vi "Named Controls Test.vi"() -> ()   [LabVIEW 2013]
uses:
  Dashboard Code/Preferences/Named Control.ctl
  Common Code/Dashboard UDP Packet.ctl
  Common Code/Dashboard UDP/Camera Controls.ctl
  Common Code/Dashboard UDP/Gyro Controls.ctl
  Common Code/Dashboard UDP/PID Params.ctl
  Common Code/Dashboard UDP/Encoder Controls.ctl
  Common Code/Dashboard UDP/Auto Shift Controls.ctl
  Common Code/Dashboard UDP/Auton Controls.ctl
  Common Code/Dashboard UDP/Shooter Controls.ctl
  Common Code/Dashboard UDP/Roller Controls.ctl
panel:
  out "Count":i32
  out "Names List":string[](array[string])
  in  "Page Index (-1 = All)":i32=-1
  out "Warnings List":string
  out "Named Controls":T1
  in  "Tab Control":enum32{"Page 0", "Page 1", "Page 2"}(tab)
  in  "Color Components":T2={"Hue"={110.0, 142.0}, "Sat"={138.0, 255.0}, "Val"={139.0, 198.0}} {"Val" scale=0.0..255.0; "Sat" scale=0.0..255.0; "Hue" scale=0.0..255.0 scale format="%#_3g"}
  in  "UDP Packet":T3={"Camera"={"Camera/View Angle X"=-1.0, "Camera/Goal Track Timeout"=-1.0, "Camera/View Angle Y"=-1.0, "Camera/Goal Exposure"=-1.0, "Camera/Vision Receive Timeout"=-1.0, "Camera/Offset 1"=-1.0, "Camera/Offset 2"=-1.0}, "Gyro"={"Gyro/Angle Tolerance"=-1.0, "Gyro/Steer Closeness Threshold"=-1.0, "Steer PID"={"max"=-1.0, "min"=-1.0, "P"=-1.0, "I"=-1.0, "D"=-1.0}, "Steer Close PID"={"max"=-1.0, "min"=-1.0, "P"=-1.0, "I"=-1.0, "D"=-1.0}}, "Encoder"={"Encoders/Reset"=FALSE, "Encoders/Omni Constant"=-1.0, "Encoders/Omni Tick Constant"=-1.0, "Encoders/Left Constant"=-1.0, "Encoders/Right Constant"=-1.0, "Encoders/Right Tick Constant"=-1.0}, "Auto Shift"={"AutoShift/Upshift Throttle Accel"=-1.0, "AutoShift/Speed Threshold"=-1.0, "AutoShift/Upshift Throttle"=-1.0, "AutoShift/Upshift Accel"=-1.0, "AutoShift/Downshift Accel"=-1.0, "AutoShift/Downshift Throttle"=-1.0, "AutoShift/Delay"=-1.0, "AutoShift/Enabled"=FALSE}, "Auton"={"Auton/Left Shoot X-Coord"=-1.0, "Auton/Right Shoot X-Coord"=-1.0, "DistDrive/Distance Stop Threshold"=0.0, "DistDrive/Max Stop Speed"=0.0, "Auton/Back Piston Time"=-1.0, "Auton/Manual Hot"=FALSE, "Auton/Manual Hot Right"=FALSE, "Default X PID"={"max"=-1.0, "min"=-1.0, "P"=-1.0, "I"=-1.0, "D"=-1.0}, "Default Y PID"={"max"=-1.0, "min"=-1.0, "P"=-1.0, "I"=-1.0, "D"=-1.0}}, "Drive/Ramp X"=-1.0, "Drive/Ramp Y"=-1.0, "Drive/Battery Cutoff"=-1.0, "Pressure/Compressor Min Voltage"=-1.0, "Pressure/Compressor Delay"=-1.0, "Controller/Strafe Correction"=FALSE, "Shooter"={"Shooter/Reset Time"=-1.0, "Shooter/Release Delay"=-1.0, "Shooter/Pressure Steady Time"=-1.0, "Shooter/Misfire Delay"=-1.0, "Shooter/Ball Settle Time"=-1.0, "Shooter/Line IR Delay"=-1.0, "Pressure/Upper PSI Time"=-1.0, "Pressure/Lower PSI Time"=-1.0, "Shooter/Punch Delay"=-1.0, "Shooter/Target Pressure"=-1.0, "Pressure/Line B"=-1.0, "Pressure/Line M"=-1.0, "Pressure/Shooter M"=-1.0, "Pressure/Shooter B"=-1.0}, "Rollers"={"Roller/Load IRs Verify Time"=-1.0, "Roller/Center IR Latch Time"=-1.0, "Roller/Speed Front"=-1.0, "Roller/Speed Back"=-1.0, "Roller/Entry Timeout"=-1.0, "Roller/To Center Timeout"=-1.0, "Roller/Sustain Time"=-1.0, "Roller/Verify Center Time"=-1.0}, "Abort"=FALSE, "Finish"=FALSE, "Shooter Halo Time"=0.0, "IR Halo Sustain Time"=0.0, "Disable Compressor"=FALSE}
  in  "HSV Filter":T12
  in  "Score Cutoff":dbl(slide)=54.248366013071895 scale=0.0..100.0
  # "Line"
  # "Shooter"
  # "Down"
  # "Up"
  # "Feet"
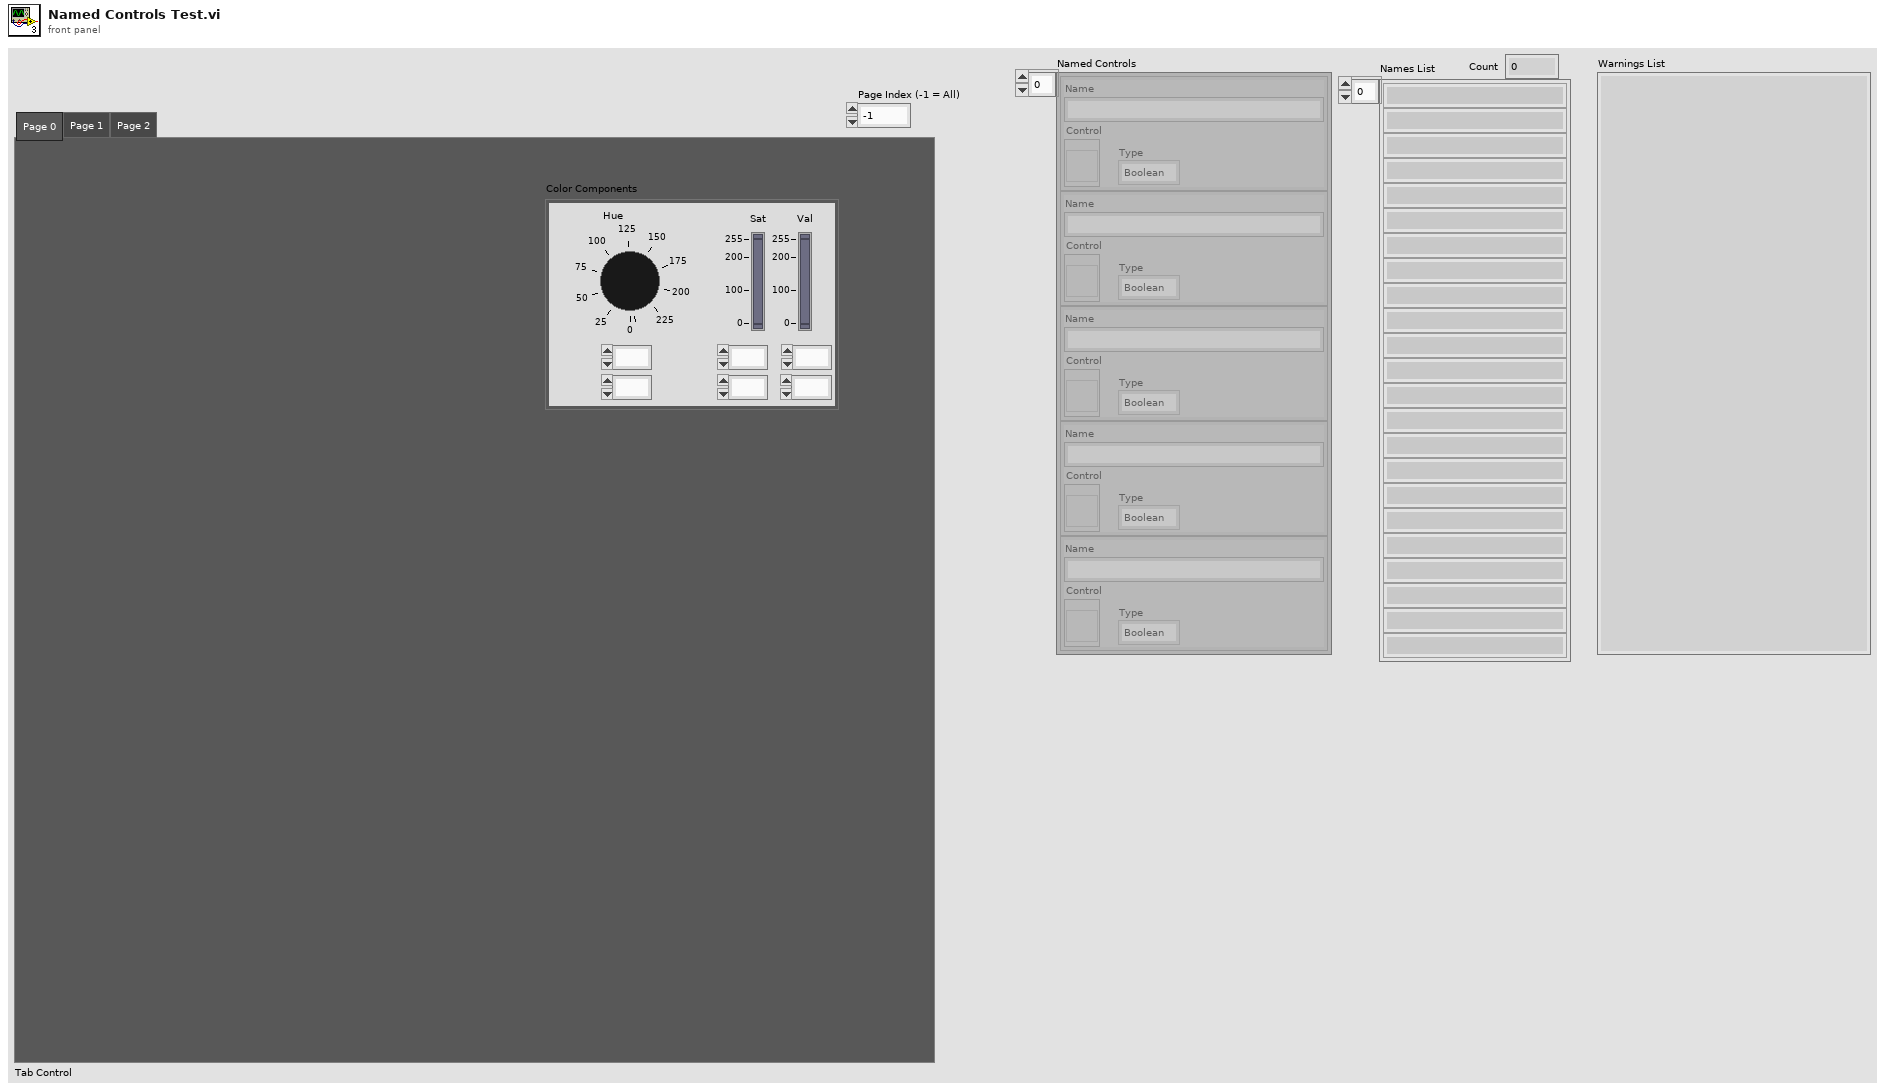
[diagram p1: front panel]
types:
  T1 = typedef "Named Control.ctl" = cluster{"Name":string, "Control":refnum<vi>, "Type":enum16{"Boolean", "Double"}}[]
  T2 = cluster{"Hue":cluster{dbl, dbl}, "Sat":cluster{dbl, dbl}, "Val":cluster{dbl, dbl}}
  T3 = typedef "Dashboard UDP Packet.ctl" = cluster{"Camera":T4, "Gyro":T5, "Encoder":T7, "Auto Shift":T8, "Auton":T9, "Drive/Ramp X":dbl, "Drive/Ramp Y":dbl, "Drive/Battery Cutoff":dbl, "Pressure/Compressor Min Voltage":dbl, "Pressure/Compressor Delay":dbl, "Controller/Strafe Correction":bool, "Shooter":T10, "Rollers":T11, "Abort":bool, "Finish":bool, "Shooter Halo Time":dbl, "IR Halo Sustain Time":dbl, "Disable Compressor":bool}
  T4 = typedef "Camera Controls.ctl" = cluster{"Camera/View Angle X":dbl, "Camera/Goal Track Timeout":dbl, "Camera/View Angle Y":dbl, "Camera/Goal Exposure":dbl, "Camera/Vision Receive Timeout":dbl, "Camera/Offset 1":dbl, "Camera/Offset 2":dbl}
  T5 = typedef "Gyro Controls.ctl" = cluster{"Gyro/Angle Tolerance":dbl, "Gyro/Steer Closeness Threshold":dbl, "Steer PID":T6, "Steer Close PID":T6}
  T6 = typedef "PID Params.ctl" = cluster{"max":dbl, "min":dbl, "P":dbl, "I":dbl, "D":dbl}
  T7 = typedef "Encoder Controls.ctl" = cluster{"Encoders/Reset":bool, "Encoders/Omni Constant":dbl, "Encoders/Omni Tick Constant":dbl, "Encoders/Left Constant":dbl, "Encoders/Right Constant":dbl, "Encoders/Right Tick Constant":dbl}
  T8 = typedef "Auto Shift Controls.ctl" = cluster{"AutoShift/Upshift Throttle Accel":dbl, "AutoShift/Speed Threshold":dbl, "AutoShift/Upshift Throttle":dbl, "AutoShift/Upshift Accel":dbl, "AutoShift/Downshift Accel":dbl, "AutoShift/Downshift Throttle":dbl, "AutoShift/Delay":dbl, "AutoShift/Enabled":bool}
  T9 = typedef "Auton Controls.ctl" = cluster{"Auton/Left Shoot X-Coord":dbl, "Auton/Right Shoot X-Coord":dbl, "DistDrive/Distance Stop Threshold":dbl, "DistDrive/Max Stop Speed":dbl, "Auton/Back Piston Time":dbl, "Auton/Manual Hot":bool, "Auton/Manual Hot Right":bool, "Default X PID":T6, "Default Y PID":T6}
  T10 = typedef "Shooter Controls.ctl" = cluster{"Shooter/Reset Time":dbl, "Shooter/Release Delay":dbl, "Shooter/Pressure Steady Time":dbl, "Shooter/Misfire Delay":dbl, "Shooter/Ball Settle Time":dbl, "Shooter/Line IR Delay":dbl, "Pressure/Upper PSI Time":dbl, "Pressure/Lower PSI Time":dbl, "Shooter/Punch Delay":dbl, "Shooter/Target Pressure":dbl, "Pressure/Line B":dbl, "Pressure/Line M":dbl, "Pressure/Shooter M":dbl, "Pressure/Shooter B":dbl}
  T11 = typedef "Roller Controls.ctl" = cluster{"Roller/Load IRs Verify Time":dbl, "Roller/Center IR Latch Time":dbl, "Roller/Speed Front":dbl, "Roller/Speed Back":dbl, "Roller/Entry Timeout":dbl, "Roller/To Center Timeout":dbl, "Roller/Sustain Time":dbl, "Roller/Verify Center Time":dbl}
  T12 = cluster{"Hue min":dbl, "Hue max":dbl, "Sat min":dbl, "Sat max":dbl, "Lum min":dbl, "Lum max":dbl}
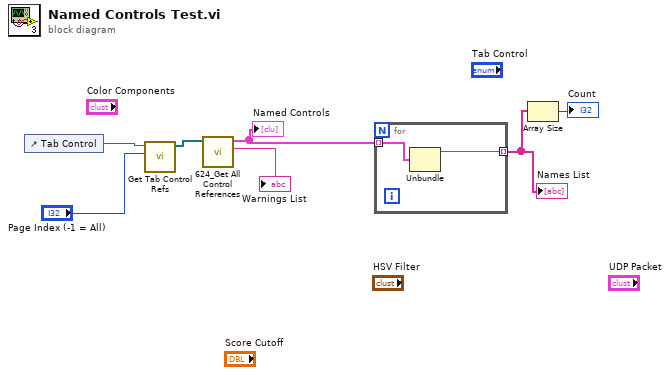
[diagram p0: block diagram]
diagram:
  n1 = control-ref of="Tab Control"() -> (w7:refnum<vi>)
  n2 = call <vilib>:"Get Tab Control Refs.vi"("Page Index"="Page Index (-1 = All)", "TabControl in"=w7) -> ("ControlsOnPage"=w6:refnum<vi>[])  [unwired: 9 in]
  n3 = call "624_Get All Control References.vi"("Controls[] in"=w6) -> ("Warnings List"=→"Warnings List":string, "Named Controls"=w4:T1)  [unwired: 8 in, 1 out]
  "Named Controls" <- w4
  n4 = for {
    tunnel: w4 -> [w9] mode=indexing
    tunnel: [w8] -> w3 mode=indexing
    n5 = Unbundle(w9) -> ("Name"=w8:string)  [unwired: 2 out]
  }
  "Names List" <- w3
  n6 = Array Size(array=w3) -> (size(s)=→"Count":i32)
